vi "PLC Test.vi"() -> ()   [LabVIEW 2020]
uses:
  DelatModbusTcp/series.ctl
  EventLogger.lvlibp/1abvi3w/vi.lib/gpm_packages/@cs/event-logger/Source/Composed Log/Types/Log Level.ctl
  EventLogger.lvlibp/1abvi3w/vi.lib/gpm_packages/@cs/event-logger/Source/Text File Sink/Configuration.ctl
  Abstract PLC Controler/Abstract PLC Controler.lvclass/Abstract PLC Controler.ctl
  DelatModbusTcp/DelatModbusTcp.lvclass
  D:/Project/Labview-Projects/General utility tool/Libraries/HslCommunication/Abstract PLC Controler/Abstract PLC Controler.lvclass
  Abstract PLC Controler/Abstract PLC Controler.lvclass
  EventLogger.lvlibp/Logger.lvclass
  EventLogger.lvlibp/1abvi3w/vi.lib/gpm_packages/@cs/event-logger/Source/Composed Log/Composed Log.lvlib
  EventLogger.lvlibp/1abvi3w/vi.lib/gpm_packages/@cs/event-logger/Source/Text File Sink/Text File Sink.lvclass
  InovanceTCP/InovanceModbusTcp.lvclass
panel:
  in  "Series":T1 items=["DVP", "AS"]
  in  "Array":dbl[](array[numeric]) format="%#_13g"
  in  "Start address":string="M12"
  out "Data":variant
  in  "length":u16
  in  "Write":bool
  in  "Read":bool
  in  "Tab Control":enum32{"InovanceModbusTcp", "Page 2"}(tab)
  in  "port":i32=502
  in  "station":u8=1
  in  "ipAddress":string="192.168.1.88"
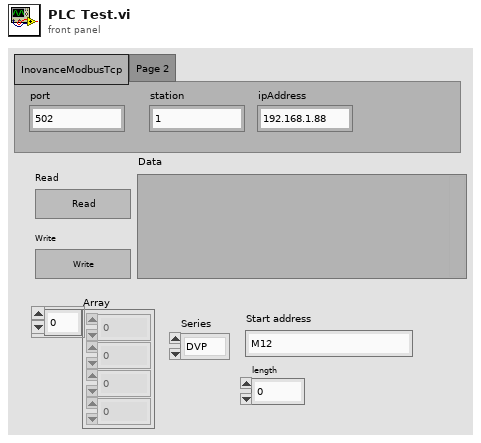
[diagram p1: front panel]
types:
  T1 = typedef "DelatModbusTcp.lvclass/series.ctl" = i32
  T2 = typedef "EventLogger.lvlibp/Text File Sink.lvclass/Configuration.ctl" = cluster{"Folder":path, "Name":string, "Extension":string, "Max Size (MB)":i64, "Timestamp Filename":bool}
  T3 = typedef "EventLogger.lvlibp/Composed Log.lvlib/Log Level.ctl" = enum16{"Debug", "Info", "Warning", "Error", "Critical"}
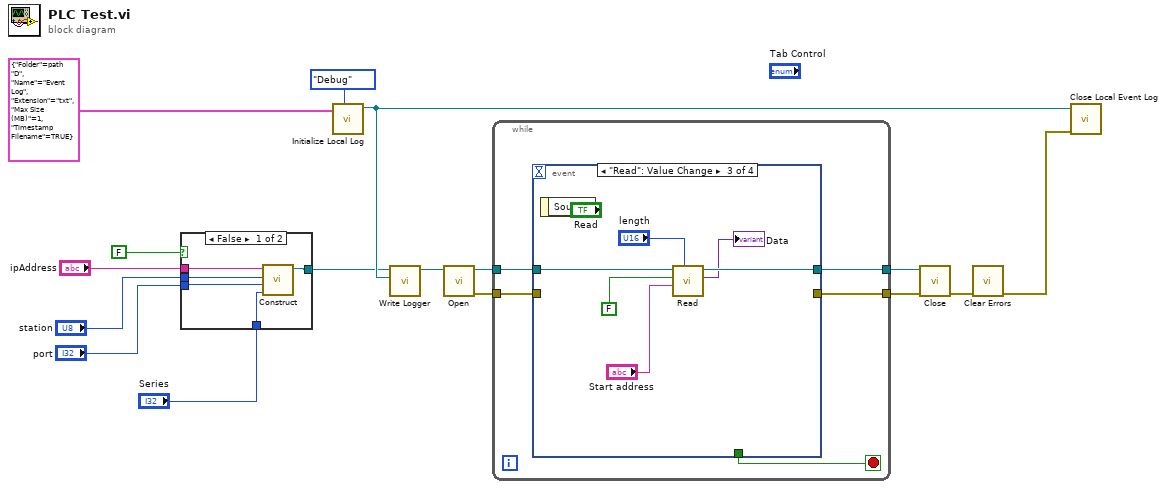
[diagram p0: block diagram]
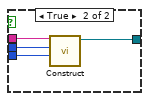
[diagram p2: hidden frame]
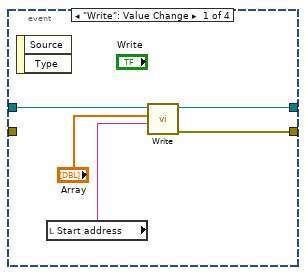
[diagram p3: hidden frame]
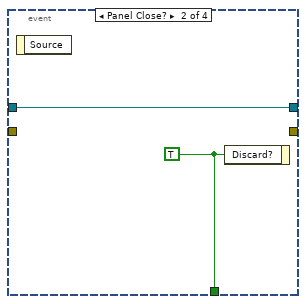
[diagram p4: hidden frame]
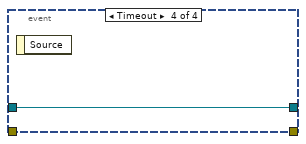
[diagram p5: hidden frame]
diagram:
  n1 = case shown="False" FALSE {
    tunnel: [w18 w24] -> w13
    tunnel: "port" -> [_ w23]
    tunnel: "station" -> [w19 w22]
    tunnel: "ipAddress" -> [w20 w21]
    tunnel: "Series" -> [w17 _]
    frame False {
      n2 = call "Construct.vi"("Series"=w17, "port"=w19, "station"=w19, "ipAddress"=w20) -> ("MelsecMcNet out"=w18:refnum<class "DelatModbusTcp.lvclass">)  [unwired: 7 in]
    }
    frame True {
      n3 = call "Construct.vi"("port"=w23, "station"=w22, "ipAddress"=w21) -> ("MelsecMcNet out"=w24:refnum<class "InovanceModbusTcp.lvclass">)  [unwired: 8 in]
    }
  }
  n4 = call "Initialize Local Log.vi"("LogLevel"=Log_Level."Debug", "Text File Configuration"=T2 {"Folder"=path "D:/", "Name"="Event Log", "Extension"="txt", "Max Size (MB)"=1, "Timestamp Filename"=TRUE}) -> ("Logger out"=w14:refnum<class "Logger.lvclass">)  [unwired: 8 in, 1 out]
  n5 = call "Write Logger.vi"("EventLogger.lvlibp:Logger.lvclass"=w14, "Abstract PLC Controler in"=w13) -> ("Abstract PLC Controler out"=w8:refnum<class "Abstract PLC Controler.lvclass">)  [unwired: 9 in]
  n6 = call-dynamic "Open.vi"("MelsecTCP in"=w8) -> ("error out"=w2:errorcluster, "MelsecTCP out"=w6:refnum<class "Abstract PLC Controler.lvclass">)  [unwired: 9 in]
  n7 = while {
    tunnel: w6 -> [w29]
    tunnel: [w28] -> w5
    tunnel: [w26] -> w4
    tunnel: w2 -> [w25]
    stop <- w27 stop-if-true
    n8 = event shown="[2] \"Read\": Value Change" {
      selector: _ -> [_ _ _ _]
      dyn-events: _ -> [_ _ _ _]
      timeout: _ -> [_ _ _ _]
      tunnel: w29 -> [w34 w35 w42 w43]
      tunnel: [w33 w35 w41 w43] -> w28
      tunnel: [_ w36 _ _] -> w27
      tunnel: [w30 _ _ _] -> w26
      tunnel: w25 -> [_ _ _ _]
      event "Write": Value Change {
        n9 = event-data() -> ()  [unwired: 1 in, 2 out]
        n10 = local read "Start address"() -> (w31:string)
        n11 = call-dynamic "Write.vi"("Start address"=w31, "Read Type"="Array", "MelsecTCP in"=w34) -> ("error out"=w30:errorcluster, "MelsecTCP out"=w33:refnum<class "Abstract PLC Controler.lvclass">)  [unwired: 7 in]
      }
      event Panel Close? {
        w36 = TRUE ("Discard?")
        n12 = event-data() -> ()  [unwired: 1 in, 1 out]
        n13 = event-data("Discard?"=w36) -> ()  [unwired: 1 in, 1 out]
      }
      event "Read": Value Change {
        n14 = event-data() -> ()  [unwired: 1 in, 1 out]
        n15 = call-dynamic "Read.vi"("length"="length", "Start address"="Start address", "Read Type"=FALSE, "MelsecTCP in"=w42) -> ("Data"=→"Data":variant, "MelsecTCP out"=w41:refnum<class "Abstract PLC Controler.lvclass">)  [unwired: 5 in, 1 out]
      }
      event Timeout {
        n16 = event-data() -> ()  [unwired: 1 in, 1 out]
      }
    }
  }
  n17 = call-dynamic "Close.vi"("error in (no error)"=w4, "MelsecTCP in"=w5) -> ("error out"=w7:errorcluster)  [unwired: 8 in, 1 out]
  n18 = call <vilib>:"Clear Errors.vi"("error in (no error)"=w7) -> ("error out"=w12:errorcluster)  [unwired: 5 in, 1 out]
  n19 = call "Close Local Event Log.vi"("error in (no error)"=w12, "Logger in"=w14) -> ()  [unwired: 8 in, 2 out]
